vi "sphere tracking settings.vi"(7 "sphere radius":u16, 10 "tracking settings":T1={"scan radius"=0, "2^16/lines per revolution"=1394, "gx"=0.0, "rtw"=0.0, "lines per revolution"=47}) -> (2 "tracking settings out":T1={"scan radius"=0, "2^16/lines per revolution"=1394, "gx"=0.0, "rtw"=0.0, "lines per revolution"=47})   [LabVIEW 2010]
uses:
  FPGA tracking/polar tracking settings.ctl
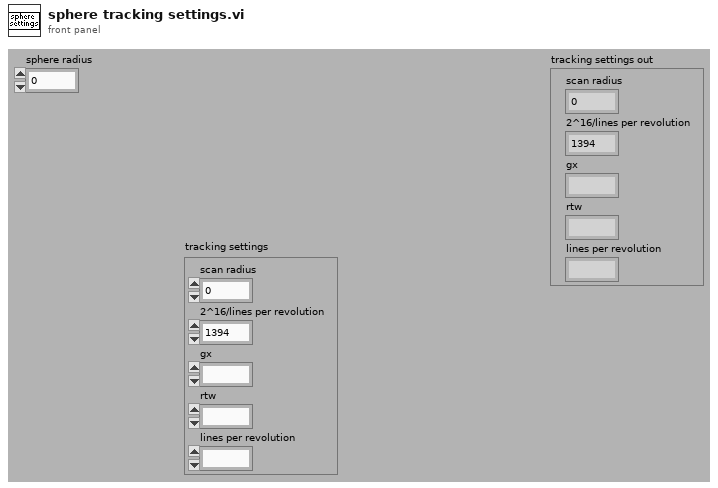
[diagram p1: front panel]
types:
  T1 = typedef "polar tracking settings.ctl" = cluster{"scan radius":u16, "2^16/lines per revolution":u16, "gx":fxp<+,16,8>, "rtw":fxp<+,16,26>, "lines per revolution":u8}
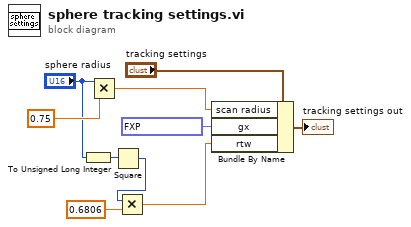
[diagram p0: block diagram]
diagram:
  n1 = To Unsigned Long Integer(number="sphere radius") -> (unsigned 32bit integer=w4:u32)
  n2 = Multiply(x="sphere radius", y=0.75) -> (x*y=w8:dbl)
  n3 = Square(x=w4) -> (x^2=w3:u32)
  n4 = Multiply(x=w3, y=0.6806) -> (x*y=w2:dbl)
  n5 = Bundle By Name(cluster="tracking settings", "scan radius"=w8, "gx"=fxp<+,16,8> 1.5546875, "rtw"=w2) -> (→"tracking settings out":T1)
